vi "Is Canceled.vi"(8 "error in":errorcluster, 11 "measure call context in":refnum<class "Measure Call Context.lvclass">) -> (0 "error out":errorcluster, 2 "is canceled?":bool, 3 "measure call context out":refnum<class "Measure Call Context.lvclass">)   [LabVIEW 2020, in "Measurement Plugin Measurement Server.lvlib" / "Measure Call Context.lvclass"]
doc: "Returns True if the measurement has been canceled by the client. The Measurement Logic VI should poll this property and immediately return when it is True."
uses:
  Measure Call Context.lvclass
  Measure Call Context.lvclass/Measure Call Context.ctl
  <vilib>/gRPC/LabVIEW gRPC Library/grpc-lvsupport-release.lvlib
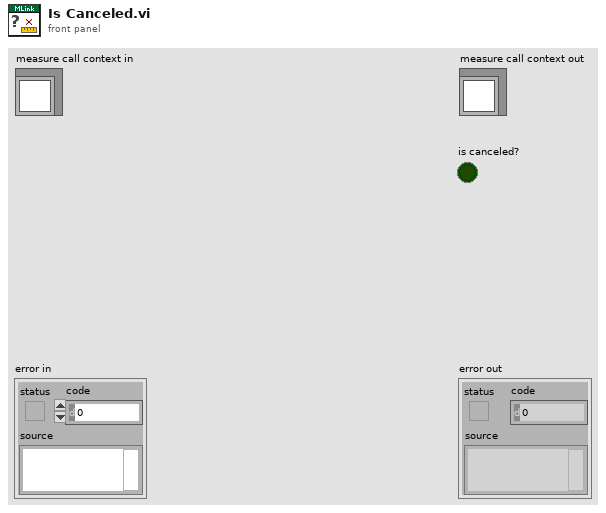
[diagram p1: front panel]
types:
  T1 = typedef "Measurement Plugin Measurement Server.lvlib/Measure Call Context.lvclass/Data.ctl" = cluster{"pin map context":T2, "gRPC ID":T3, "measurement service":refnum<class "IMeasurement Service.lvclass">, "measurement plugin service":refnum<class "Measurement Plugin Service.lvclass">, "reserved session infos":set{T4}}
  T2 = typedef "Measurement Plugin Measurement Server.lvlib/Pin Map Context.ctl" = cluster{"pin map id":string, "sites":i32[]}
  T3 = typedef "grpc-lvsupport-release.lvlib/grpcId.ctl" = u64
  T4 = typedef "MeasurementLink Session Management Client.lvlib/ni_measurementlink_sessionmanagement_v1_SessionInformation.ctl" = cluster{"session":T5, "resource_name":string, "channel_list":string, "instrument_type_id":string, "session_exists":bool, "channel_mappings":T6[]}
  T5 = typedef "MeasurementLink Session Management Client.lvlib/nidevice_grpc_Session.ctl" = cluster{"name":string}
  T6 = typedef "MeasurementLink Session Management Client.lvlib/ni_measurementlink_sessionmanagement_v1_ChannelMapping.ctl" = cluster{"pin_or_relay_name":string, "site":i32, "channel":string, "multiplexer_resource_name":string, "multiplexer_route":string}
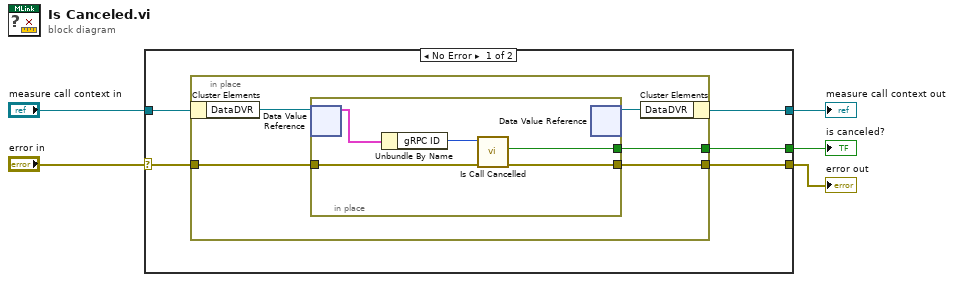
[diagram p0: block diagram]
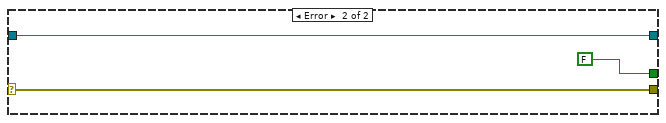
[diagram p2: hidden frame]
diagram:
  n1 = case shown="No Error" "error in" {
    selector: "error in" -> [w9 w23]
    tunnel: [w8 w23] -> w4
    tunnel: [w6 w22] -> w2
    tunnel: "measure call context in" -> [w7 w22]
    tunnel: [w10 FALSE ("Is Cancelled")] -> w1
    frame No Error {
      n2 = in-place {
        in-place-border: [w15] -> w10
        in-place-border: w9 -> [w14]
        in-place-border: [w13] -> w8
        n3 = in-place-cluster #1(w7) -> ("DataDVR"=w12:refnum<data-value>)
        n4 = in-place {
          in-place-border: [w20] -> w15
          in-place-border: w14 -> [w19]
          in-place-border: [w18] -> w13
          n5 = in-place-dvr #2(w12) -> (w17:T1)  [unwired: 1 out]
          n6 = Unbundle By Name(w17) -> ("gRPC ID"=w16:T3)
          n7 = call <vilib>:"Is Call Cancelled.vi"("error in"=w19, "gRPCid in"=w16) -> ("error out"=w18:errorcluster, "Is Cancelled"=w20:bool)  [unwired: 7 in, 1 out]
          n8 = in-place-dvr #2() -> (w11:refnum<data-value>)  [unwired: 1 in, 1 out]
        }
        n9 = in-place-cluster #1("DataDVR"=w11) -> (w6:refnum<class "Measure Call Context.lvclass">)
      }
    }
    frame Error {
    }
  }
  "error out" <- w4
  "measure call context out" <- w2
  "is canceled?" <- w1
